vi "Cryo-Con Set T.vi"(8 "error in (no error)":errorcluster, 10 "Set T":dbl=2.0, 11 "VISA Resource Name":refnum<visa-resource-name>) -> (0 "error out":errorcluster, 3 "VISA Resource Name Out":refnum<visa-resource-name>)   [LabVIEW 2019]
panel:
  out "resulting string":string
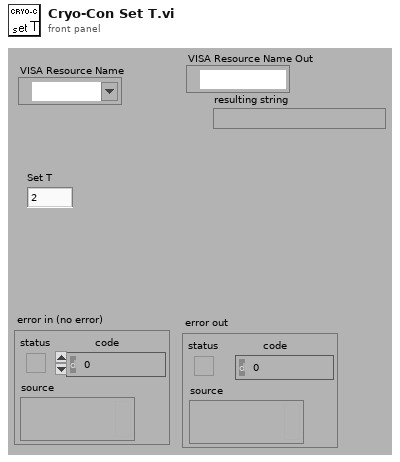
[diagram p1: front panel]
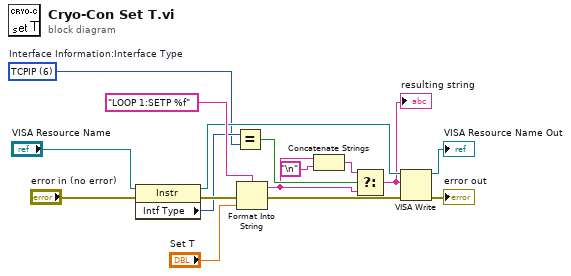
[diagram p0: block diagram]
diagram:
  w6 = u16 6 items=["GPIB"=1, "VXI"=2, "GPIB-VXI"=3, "Serial"=4, "PXI"=5, "TCPIP"=6, "USB"=7, "FireWire"=9]  # Interface Information:Interface Type
  n1 = property class="Instr"(reference="VISA Resource Name", error in="error in (no error)") -> (reference out=w8:refnum<visa-resource-name>, error out=w10:errorcluster, "Intf Type"=w7:u16)
  n2 = Equal?(x=w7, y=w6) -> (x = y?=w5:bool)
  n3 = Format Into String(format string="LOOP 1:SETP %f", error in=w10, "Set T") -> (resulting string=w2:string, error out=w13:errorcluster)  [unwired: 1 in]
  n4 = Concatenate Strings(w2, "\n") -> (w3:string)
  n5 = Select(t=w3, s=w5, f=w2) -> (s? t:f=w1:string)
  "resulting string" <- w1
  n6 = VISA Write(VISA resource name=w8, write buffer=w1, error in (no error)=w13) -> (VISA resource name out=→"VISA Resource Name Out":refnum<visa-resource-name>, error out=→"error out":errorcluster)  [unwired: 1 out]
